vi "Read From File.vi"(8 "error in (no error)":errorcluster, 11 "file path":path) -> (0 "error out":errorcluster, 2 "analog generation":T1={"output rate"=0.0, "range"=0.0, "terminal configuration"=enum."Pseudodifferential", "output impedance"=0.0, "common mode offset"=0.0, "pure tone mode"=FALSE}, 5 "file exists?":bool)   [LabVIEW 2021, in "Analog Gen Settings.lvlib"]
uses:
  Analog Gen Settings.lvlib
  service/generation/controls/analog output settings.ctl
  service/generation/controls/terminal configuration.ctl
  analog output settings_json.ctl
  service/generation/controls/AudioGenTypeDefs.lvlib
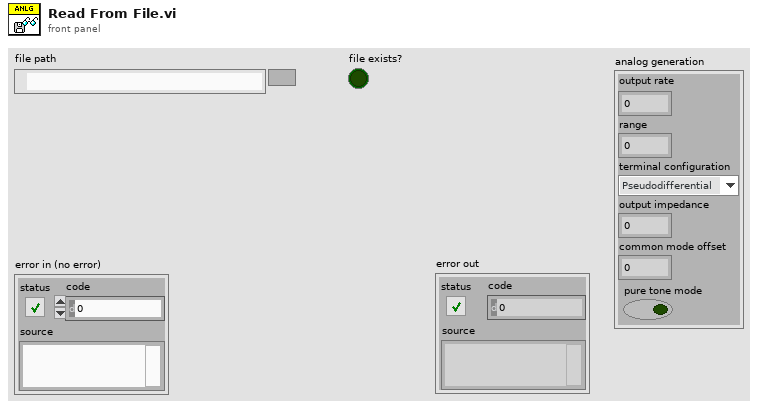
[diagram p1: front panel]
types:
  T1 = typedef "AudioGenTypeDefs.lvlib/analog output settings.ctl" = cluster{"output rate":dbl, "range":dbl, "terminal configuration":T2, "output impedance":dbl, "common mode offset":dbl, "pure tone mode":bool}
  T2 = typedef "AudioGenTypeDefs.lvlib/terminal configuration.ctl" = enum32{"Default", "RSE", "Differential", "Pseudodifferential"}
  T3 = typedef "Analog Gen Settings.lvlib/analog output settings_json.ctl" = cluster{"output rate":dbl, "range":dbl, "terminal configuration":string, "output impedance":dbl, "common mode offset":dbl, "pure tone mode":bool}
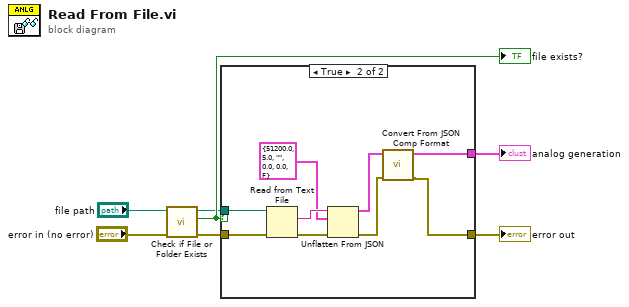
[diagram p0: block diagram]
diagram:
  n1 = call <vilib>:"Check if File or Folder Exists.vi"("error in (no error)"="error in (no error)", "path"="file path") -> ("error out"=w6:errorcluster, "file or folder exists?"=w5:bool, "dup path"=w4:path)  [unwired: 7 in]
  "file exists?" <- w5
  n2 = case shown="True" w5 {
    tunnel: w6 -> [w8 w16]
    tunnel: w4 -> [_ w17]
    tunnel: [_ w12] -> w1
    tunnel: [w8 w10] -> w2
    frame False {
      # "no file found"
    }
    frame True {
      n3 = Read from Text File(file (use dialog)=w17, error in=w16) -> (text=w14:string, error out=w15:errorcluster)  [unwired: 2 in, 2 out]
      n4 = Unflatten From JSON(JSON string=w14, type and defaults=T3 {"output rate"=51200.0, "range"=5.0, "terminal configuration"="", "output impedance"=0.0, "common mode offset"=0.0, "pure tone mode"=FALSE} ("output settings"), error in (no error)=w15) -> (value=w13:T3, error out=w11:errorcluster)  [unwired: 4 in]
      n5 = call "Convert From JSON Comp Format.vi"("output settings JSON"=w13, "error in (no error)"=w11) -> ("error out"=w10:errorcluster, "output settings"=w12:T1)  [unwired: 8 in]
    }
  }
  "error out" <- w2
  "analog generation" <- w1
